vi "Direct.vi"(7 "Actor in":refnum<class "Actor.lvclass">, 9 "Error":errorcluster, 10 "Actor":refnum<class "Actor.lvclass">) -> (0 "Error out":errorcluster, 5 "Actor out":refnum<class "Actor.lvclass">)   [LabVIEW 2025, in "jettl.lvlib" / "Finish Msg.lvlib"]
uses:
  Finish Msg.lvlib
  Actor/Actor/Actor.lvclass
  Finish Msg/Finish Msg.lvclass
  Actor/Actor.lvlib
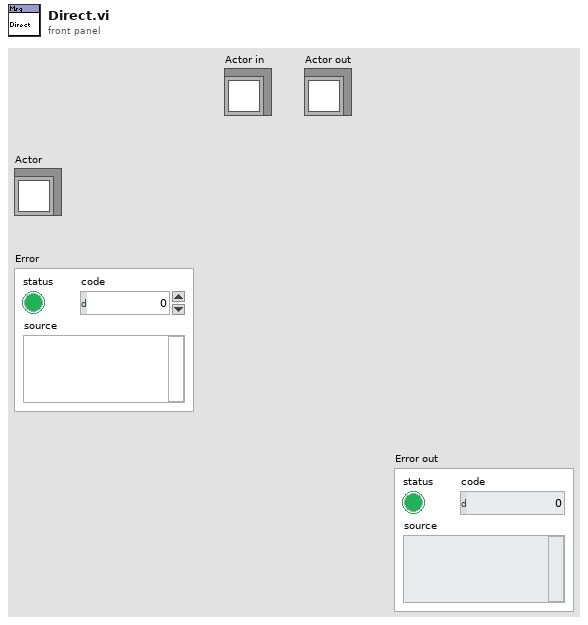
[diagram p1: front panel]
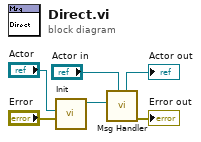
[diagram p0: block diagram]
diagram:
  n1 = call "Init.vi"("Error"="Error", "Actor"="Actor") -> ("Finish Msg out"=w3:refnum<class "Finish Msg.lvclass">)  [unwired: 9 in]
  n2 = call "Msg Handler.vi"("Actor in"="Actor in", "Msg"=w3) -> ("Error out"=→"Error out":errorcluster, "Actor out"=→"Actor out":refnum<class "Actor.lvclass">)  [unwired: 8 in]
